vi "Tester.vi"() -> ()   [LabVIEW 2024, in "Tester.lvlib"]
uses:
  Tester.lvlib
  Tests/tests--enum.ctl
  <vilib>/Utility/High Resolution Relative Seconds.vi
  <vilib>/Analysis/baseanly.llb/Std Deviation and Variance.vi
panel:
  in  "Packet Size":i32=5000 caption="Numeric"
  in  "Copy Data":bool
  in  "Copy Results":bool
  out "Tests":T1[](array[typedef])
  out "Test Results":dbl[][](array[numeric]) format="%_4p"
  out "Raw Data":dbl[][](graph)
  out "Result":string[](array[string])
  in  "Data Size":i32=12000 caption="Numeric"
  in  "Test":T1
  in  "Reset":bool
  in  "Run":bool
  in  "Num of Calls":i32=1000 caption="Numeric"
  # "Mean (s)"
  # "StDev"
  # "Max (s)"
  # "Min (s)"
  # "Always wire up the final output to keep the compiler from being too smart thinking the data's never used so why bother"
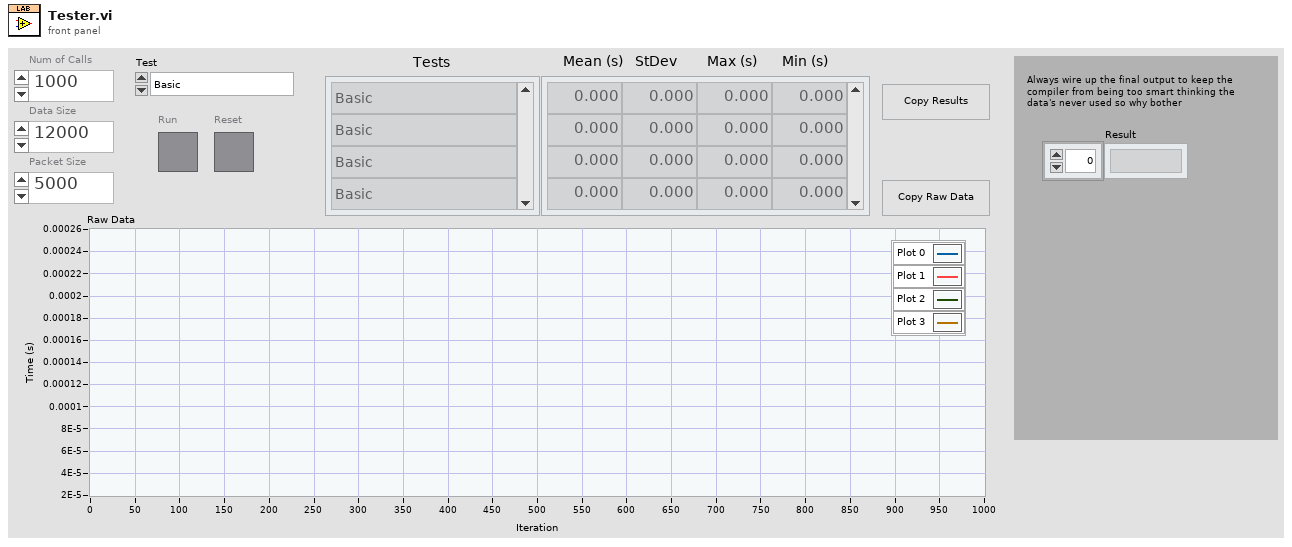
[diagram p1: front panel]
types:
  T1 = typedef "Tester.lvlib/tests--enum.ctl" = enum16{"Basic", "Pre-Allocated", "Packet-Type Case", "No IPE"}
  T2 = typedef "Tester.lvlib/test_data--cluster.ctl" = cluster{"data":dbl[], "encoded packets":string[], "packet size":i32, "packetized data":T3[]}
  T3 = typedef "Tester.lvlib/packetized_data--cluster.ctl" = cluster{"Type":enum16{"Full Set", "Last Set"}, "Data":dbl[], "Encoded":string}
  T4 = typedef "test_data--cluster.ctl" = cluster{"Tests":T1[], "results":dbl[][], "raw_data":dbl[][]}
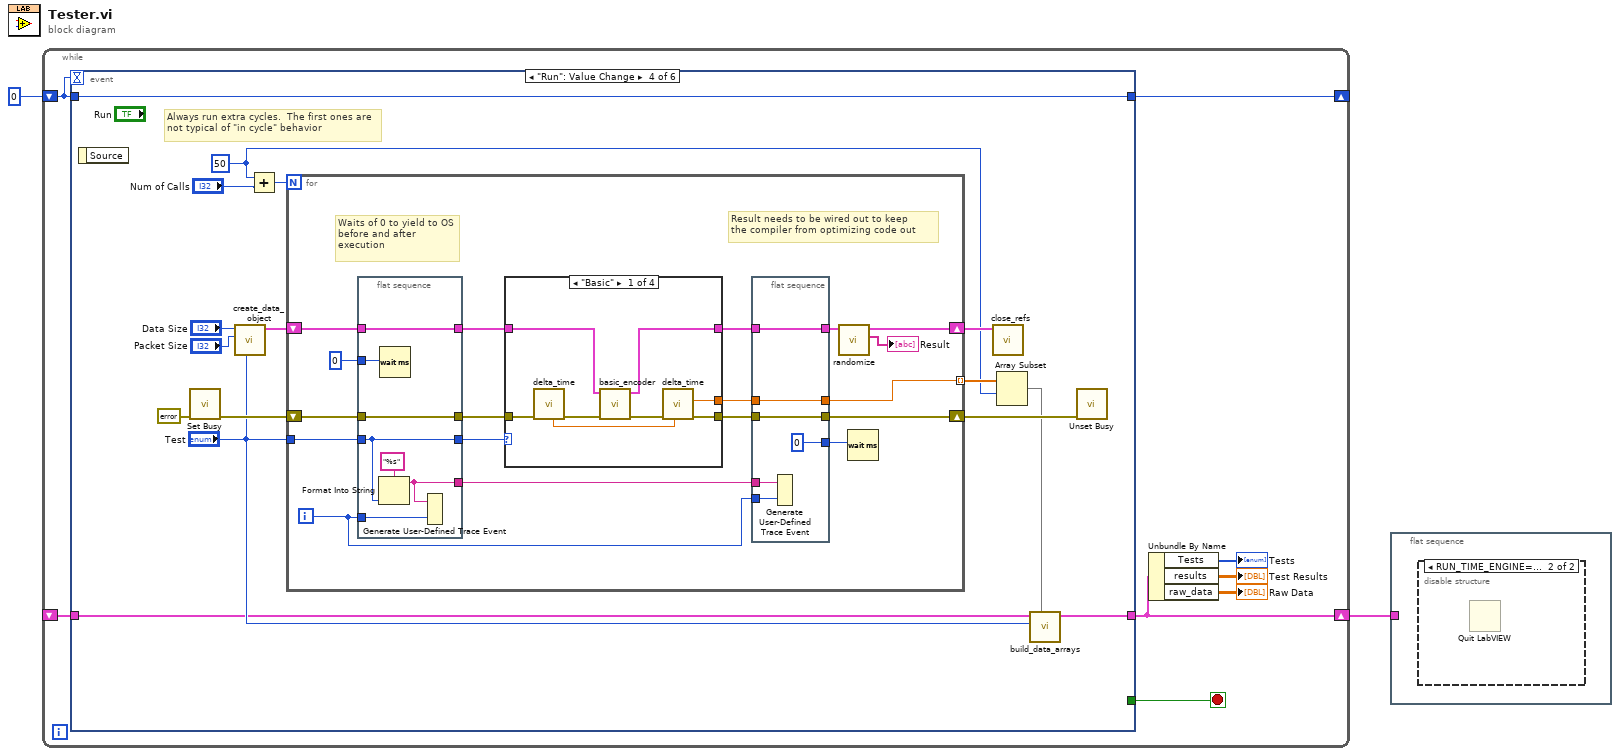
[diagram p0: block diagram]
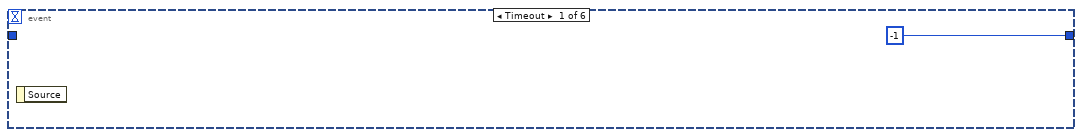
[diagram p3: hidden frame]
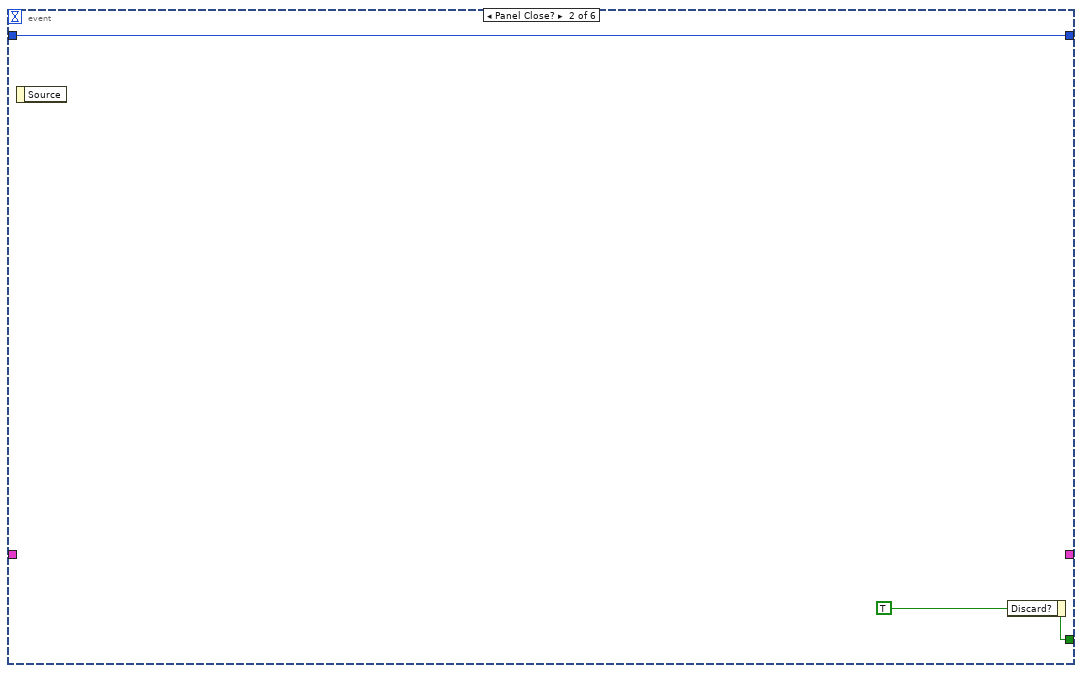
[diagram p4: hidden frame]
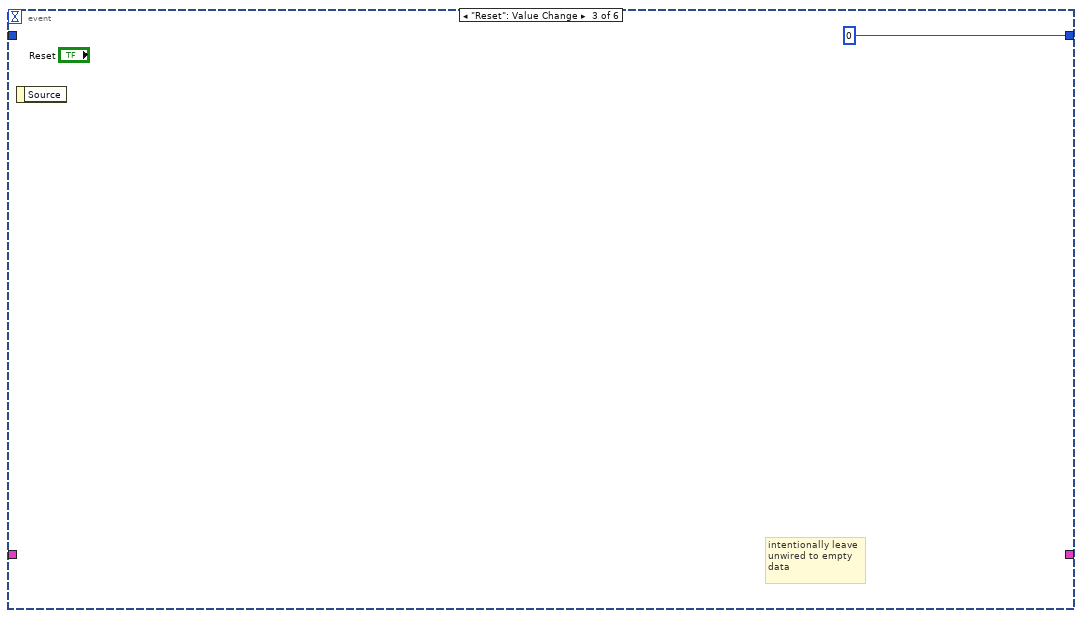
[diagram p5: hidden frame]
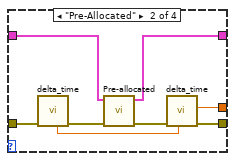
[diagram p6: hidden frame]
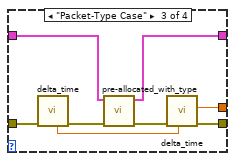
[diagram p7: hidden frame]
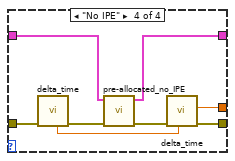
[diagram p8: hidden frame]
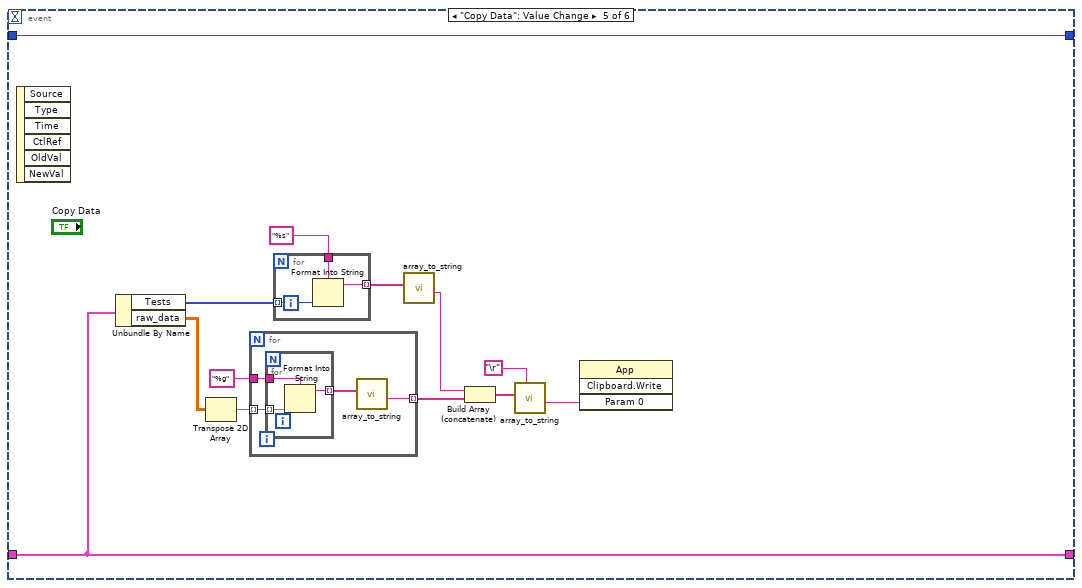
[diagram p9: hidden frame]
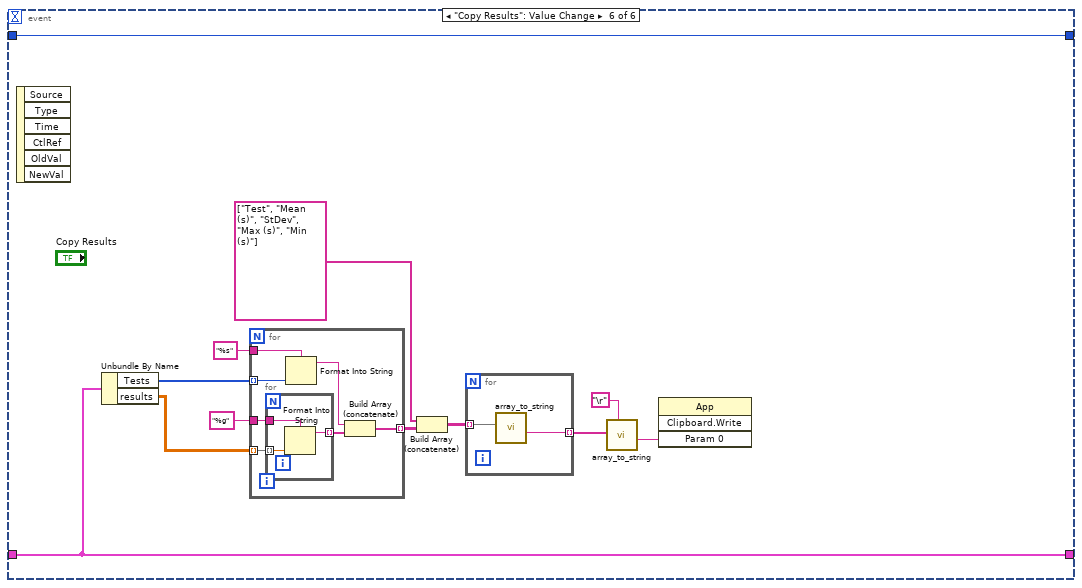
[diagram p10: hidden frame]
diagram:
  n1 = while {
    shift-right: [w9] -> _
    shift-left: 0 -> [w10]
    shift-right: [w6] -> w1
    shift-left: _ -> [w7]
    stop <- w8 stop-if-true
    n2 = event shown="[3] \"Run\": Value Change" {
      selector: _ -> [_ _ _ _ _ _]
      dyn-events: _ -> [_ _ _ _ _ _]
      timeout: w10 -> [_ _ _ _ _ _]
      tunnel: w10 -> [_ w13 _ w30 w106 w128]
      tunnel: [-1 w13 0 w30 w106 w128] -> w9
      tunnel: [_ w12 _ _ _ _] -> w8
      tunnel: w7 -> [_ _ _ w15 w96 w119]
      tunnel: [_ _ _ w16 w96 w119] -> w6
      event Timeout {
        n3 = event-data() -> ()  [unwired: 1 in, 1 out]
      }
      event Panel Close? {
        w12 = TRUE ("Discard?")
        n4 = event-data() -> ()  [unwired: 1 in, 1 out]
        n5 = event-data("Discard?"=w12) -> ()  [unwired: 1 in, 1 out]
      }
      event "Reset": Value Change {
        # "intentionally leave\nunwired to empty\ndata"
        n6 = event-data() -> ()  [unwired: 1 in, 1 out]
      }
      event "Run": Value Change {
        w21 = 50 ("x")
        # "Always run extra cycles.  The first ones are not typical of \"in cycle\" behavior"
        n7 = event-data() -> ()  [unwired: 1 in, 1 out]
        n8 = call <vilib>:"Set Busy.vi"("error in (no error)"=errorcluster {"status"=FALSE, "code"=0, "source"=""}) -> ("error out"=w27:errorcluster)  [unwired: 9 in, 1 out]
        n9 = call "create_data_object.vi"("Test"="Test", "packet size"="Packet Size", "data size"="Data Size") -> ("Test Data"=w28:T2)  [unwired: 8 in]
        n10 = Add(x=w21, y="Num of Calls") -> (x+y=w22:i32)
        n11 = for {
          N: w22 -> [_]
          shift-right: [w36] -> w24
          shift-left: w28 -> [w46]
          shift-right: [w43] -> w26
          shift-left: w27 -> [w47]
          tunnel: "Test" -> [w48]
          tunnel: [w40] -> w25 mode=indexing
          i -> [w42]
          # "Waits of 0 to yield to OS before and after execution"
          # "Result needs to be wired out to keep\nthe compiler from optimizing code out"
          n12 = flat-sequence {
            tunnel: [w90] -> w41
            tunnel: w48 -> [w90]
            tunnel: w42 -> [w91]
            tunnel: [w93] -> w45
            tunnel: w47 -> [w93]
            tunnel: w46 -> [w92]
            tunnel: [w92] -> w38
            tunnel: [w88] -> w33
            tunnel: u32 0 -> [w87]
            frame #0 {
              n13 = Format Into String(format string="%s", w90) -> (resulting string=w88:string)  [unwired: 2 in, 1 out]
              n14 = Wait (ms)(milliseconds to wait=w87) -> ()  [unwired: 1 out]
              n15 = Generate User-Defined Trace Event(1:w91, 2:w88) -> ()
            }
          }
          n16 = case shown="\"Basic\"" w41 {
            tunnel: w45 -> [w62 w70 w78 w86]
            tunnel: [w60 w68 w76 w84] -> w44
            tunnel: [w59 w67 w75 w83] -> w39
            tunnel: w38 -> [w56 w64 w72 w80]
            tunnel: [w55 w63 w71 w79] -> w37
            frame "Basic" {
              n17 = call "delta_time.vi"("error in (no error)"=w62) -> ("error out"=w58:errorcluster, "Time out"=w61:dbl)  [unwired: 8 in, 1 out]
              n18 = call "basic_encoder.vi"("error in (no error)"=w58, "Test Data in"=w56) -> ("error out"=w57:errorcluster, "Test Data out"=w55:T2)  [unwired: 8 in]
              n19 = call "delta_time.vi"("Time in"=w61, "error in (no error)"=w57) -> ("error out"=w60:errorcluster, "Delta Time"=w59:dbl)  [unwired: 7 in, 1 out]
            }
            frame "Pre-Allocated" {
              n20 = call "delta_time.vi"("error in (no error)"=w70) -> ("error out"=w66:errorcluster, "Time out"=w69:dbl)  [unwired: 8 in, 1 out]
              n21 = call "Pre-allocated.vi"("error in (no error)"=w66, "Test Data in"=w64) -> ("error out"=w65:errorcluster, "Test Data out"=w63:T2)  [unwired: 8 in]
              n22 = call "delta_time.vi"("Time in"=w69, "error in (no error)"=w65) -> ("error out"=w68:errorcluster, "Delta Time"=w67:dbl)  [unwired: 7 in, 1 out]
            }
            frame "Packet-Type Case" {
              n23 = call "delta_time.vi"("error in (no error)"=w78) -> ("error out"=w74:errorcluster, "Time out"=w77:dbl)  [unwired: 8 in, 1 out]
              n24 = call "pre-allocated_with_type.vi"("error in (no error)"=w74, "Test Data in"=w72) -> ("error out"=w73:errorcluster, "Test Data out"=w71:T2)  [unwired: 8 in]
              n25 = call "delta_time.vi"("Time in"=w77, "error in (no error)"=w73) -> ("error out"=w76:errorcluster, "Delta Time"=w75:dbl)  [unwired: 7 in, 1 out]
            }
            frame "No IPE" {
              n26 = call "delta_time.vi"("error in (no error)"=w86) -> ("error out"=w82:errorcluster, "Time out"=w85:dbl)  [unwired: 8 in, 1 out]
              n27 = call "pre-allocated_no_IPE.vi"("error in (no error)"=w82, "Test Data in"=w80) -> ("error out"=w81:errorcluster, "Test Data out"=w79:T2)  [unwired: 8 in]
              n28 = call "delta_time.vi"("Time in"=w85, "error in (no error)"=w81) -> ("error out"=w84:errorcluster, "Delta Time"=w83:dbl)  [unwired: 7 in, 1 out]
            }
          }
          n29 = flat-sequence {
            tunnel: w42 -> [w54]
            tunnel: [w53] -> w43
            tunnel: w44 -> [w53]
            tunnel: w37 -> [w52]
            tunnel: [w52] -> w35
            tunnel: [w51] -> w40
            tunnel: w39 -> [w51]
            tunnel: w33 -> [w50]
            tunnel: [u32 0] -> w32
            frame #0 {
              n30 = Generate User-Defined Trace Event(1:w54, 2:w50) -> ()
            }
          }
          n31 = call "randomize.vi"("Test Data in"=w35) -> ("encoded packets"=→"Result":string[], "Test Data out"=w36:T2)  [unwired: 9 in]
          n32 = Wait (ms)(milliseconds to wait=w32) -> ()  [unwired: 1 out]
        }
        n33 = call "close_refs.vi"("Test Data in"=w24) -> ()  [unwired: 11 in]
        n34 = Array Subset(array=w25, index=w21) -> (w18:dbl[])  [unwired: 1 in]
        n35 = call "build_data_arrays.vi"("last_test"=w18, "Test"="Test", "test_data in"=w15) -> ("test_data out"=w16:T4)  [unwired: 8 in]
        n36 = call <vilib>:"Unset Busy.vi"("error in (no error)"=w26) -> ()  [unwired: 10 in, 1 out]
      }
      event "Copy Data": Value Change {
        n37 = event-data() -> ()  [unwired: 1 in, 6 out]
        n38 = Unbundle By Name(w96) -> ("Tests"=w94:T1[], "raw_data"=w95:dbl[][])
        n39 = Transpose 2D Array(2D array=w95) -> (transposed array=w100:dbl[][])
        n40 = for {
          tunnel: w100 -> [w108] mode=indexing
          tunnel: [w110] -> w104 mode=indexing
          tunnel: "%g" -> [w107]
          n41 = for {
            tunnel: [w113] -> w109 mode=indexing
            tunnel: w108 -> [w111] mode=indexing
            tunnel: w107 -> [w112]
            n42 = Format Into String(format string=w112, w111) -> (resulting string=w113:string)  [unwired: 2 in, 1 out]
          }
          n43 = call "array_to_string.vi"("Array of Strings"=w109) -> ("delimited string"=w110:string)  [unwired: 10 in]
        }
        n44 = for {
          tunnel: "%s" -> [w116]
          tunnel: [w115] -> w98 mode=indexing
          tunnel: w94 -> [w114] mode=indexing
          n45 = Format Into String(format string=w116, w114) -> (resulting string=w115:string)  [unwired: 2 in, 1 out]
        }
        n46 = call "array_to_string.vi"("Array of Strings"=w98) -> ("delimited string"=w97:string)  [unwired: 10 in]
        n47 = Build Array (concatenate)(w97, w104) -> (w103:string[])
        n48 = call "array_to_string.vi"("delimiter (Tab)"="\r", "Array of Strings"=w103) -> ("delimited string"=w101:string)  [unwired: 9 in]
        n49 = invoke class="App" method="Clipboard.Write"("Param 0"=w101) -> ()  [unwired: 3 in, 4 out]
      }
      event "Copy Results": Value Change {
        n50 = event-data() -> ()  [unwired: 1 in, 6 out]
        n51 = Unbundle By Name(w119) -> ("Tests"=w118:T1[], "results"=w117:dbl[][])
        n52 = for {
          tunnel: [w133] -> w127 mode=indexing
          tunnel: "%g" -> [w137]
          tunnel: "%s" -> [w136]
          tunnel: w118 -> [w132] mode=indexing
          tunnel: w117 -> [w131] mode=indexing
          n53 = for {
            tunnel: [w140] -> w135 mode=indexing
            tunnel: w137 -> [w139]
            tunnel: w131 -> [w138] mode=indexing
            n54 = Format Into String(format string=w139, w138) -> (resulting string=w140:string)  [unwired: 2 in, 1 out]
          }
          n55 = Format Into String(format string=w136, w132) -> (resulting string=w134:string)  [unwired: 2 in, 1 out]
          n56 = Build Array (concatenate)(w134, w135) -> (w133:string[])
        }
        n57 = Build Array (concatenate)(string[] ["Test", "Mean (s)", "StDev", "Max (s)", "Min (s)"], w127) -> (w121:string[][])
        n58 = for {
          tunnel: w121 -> [w130] mode=indexing
          tunnel: [w129] -> w120 mode=indexing
          n59 = call "array_to_string.vi"("Array of Strings"=w130) -> ("delimited string"=w129:string)  [unwired: 10 in]
        }
        n60 = call "array_to_string.vi"("delimiter (Tab)"="\r", "Array of Strings"=w120) -> ("delimited string"=w125:string)  [unwired: 9 in]
        n61 = invoke class="App" method="Clipboard.Write"("Param 0"=w125) -> ()  [unwired: 3 in, 4 out]
      }
    }
    n62 = Unbundle By Name(w6) -> ("Tests"=→"Tests":T1[], "results"=→"Test Results":dbl[][], "raw_data"=→"Raw Data":dbl[][])
  }
  n63 = flat-sequence {
    tunnel: w1 -> [_]
    frame #0 {
      n64 = disable-structure shown="RUN_TIME_ENGINE==True" {
        frame condition #0 (active) {
        }
        frame condition #1 {
          n65 = Quit LabVIEW() -> ()  [unwired: 1 in]
        }
      }
    }
  }
